vi "Aula 3 17_08 While_For.vi"() -> ()   [LabVIEW 2020]
panel:
  out "Seleção":dbl
  in  "T/F":bool
  in  "milliseconds to wait 2":u32=300
  out "Interação atual":i16
  in  "Num de interações":i64
  out "Numeric 4":dbl
  in  "Numeric 3":dbl
  in  "Numeric 2":dbl
  in  "milliseconds to wait":u32=300
  out "Numeric":i32
  in  "Stop Button":bool
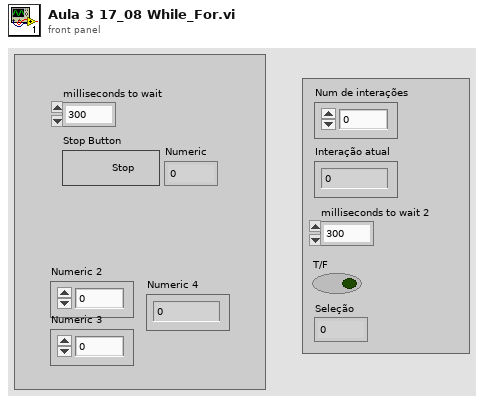
[diagram p1: front panel]
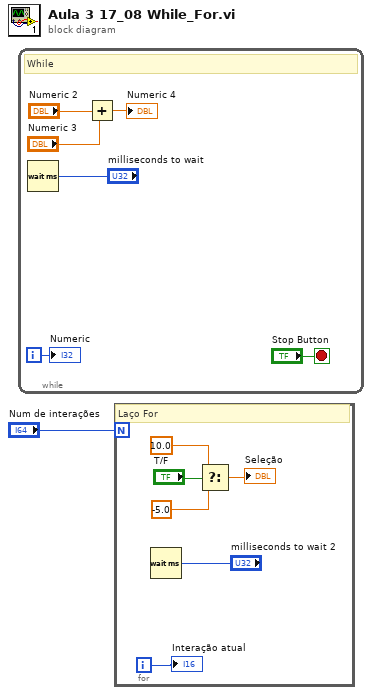
[diagram p0: block diagram]
diagram:
  n1 = while {
    i -> [w6]
    stop <- "Stop Button" stop-if-true
    # "While"
    n2 = Wait (ms)(milliseconds to wait="milliseconds to wait") -> ()  [unwired: 1 out]
    n3 = Add(x="Numeric 2", y="Numeric 3") -> (x+y=→"Numeric 4":dbl)
    "Numeric" <- w6
  }
  n4 = for {
    N: "Num de interações" -> [_]
    i -> [w13]
    # "Laço For"
    n5 = Wait (ms)(milliseconds to wait="milliseconds to wait 2") -> ()  [unwired: 1 out]
    n6 = Select(t=10.0 ("s? t:f"), s="T/F", f=-5.0 ("s? t:f")) -> (s? t:f=→"Seleção":dbl)
    "Interação atual" <- w13
  }
